vi "Post-Setup Actors.vi"(7 "Actor in":refnum<class "Actor.lvclass">) -> (2 "Post-Setup Actors":refnum<class "Actor.lvclass">[](array[class]))   [LabVIEW 2020, in "jettl.lvlib" / "Read Self Attributes.lvlib"]
uses:
  Read Self Attributes.lvlib
  Actor/Actor.lvclass
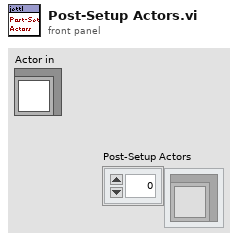
[diagram p1: front panel]
types:
  T1 = typedef "jettl.lvlib/Attributes.ctl" = cluster{"Unified Layer":T2, "Edge Layers":refnum<class "Actor.lvclass">[], "Core Layers":refnum<class "Actor.lvclass">[], "Root":bool, "Alias":string, "Transport":refnum<class "Transport.lvclass">, "UID":i32, "This VI":refnum<vi>, "Post-Setup Layers":refnum<class "Actor.lvclass">[]}
  T2 = typedef "jettl.lvlib/Layer.ctl" = cluster{"Msgs":T3, "Msg Names":T4, "Leaf":bool, "Index":i32, "Name":string}
  T3 = typedef "jettl.lvlib/Msgs.ctl" = set{refnum<class "Msg.lvclass">}
  T4 = typedef "jettl.lvlib/Msg Names.ctl" = set{string}
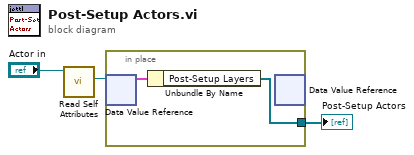
[diagram p0: block diagram]
diagram:
  n1 = call-dynamic "Read Self Attributes.vi"("Actor in"="Actor in") -> ("Self Attributes"=w2:refnum<data-value>)  [unwired: 10 in]
  n2 = in-place {
    in-place-border: [w4] -> w1
    n3 = in-place-dvr #1(w2) -> (w5:T1)  [unwired: 1 out]
    n4 = Unbundle By Name(w5) -> ("Post-Setup Layers"=w4:refnum<class "Actor.lvclass">[])
    n5 = in-place-dvr #1() -> ()  [unwired: 1 in, 2 out]
  }
  "Post-Setup Actors" <- w1
